vi "Resistance Configuration.vi"(8 "error in (no error)":errorcluster, 10 "Resistance Range":T1, 11 "VISA resource name":refnum<visa-resource-name>) -> (0 "error out":errorcluster, 3 "VISA resource name out":refnum<visa-resource-name>)   [LabVIEW 2015, in "Keysight U1252.lvlib"]
uses:
  <instrlib>/Keysight U1252/Keysight U1252.lvlib
  <instrlib>/Keysight U1252/Controls/Resistance Range.ctl
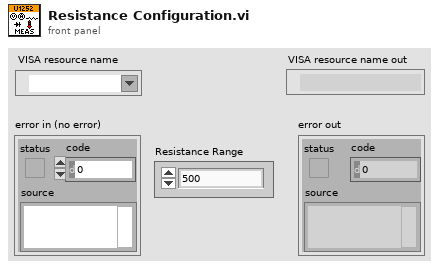
[diagram p1: front panel]
types:
  T1 = typedef "Keysight U1252.lvlib/Resistance Range.ctl" = enum16{"500", "5k", "50k", "500k", "5M", "50M", "500M", "Auto"}
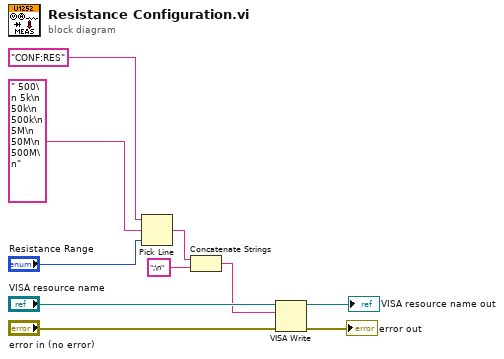
[diagram p0: block diagram]
diagram:
  n1 = Pick Line(string ("")="CONF:RES", multi-line string=" 500\n 5k\n 50k\n 500k\n 5M\n 50M\n 500M\n", line index="Resistance Range") -> (output string=w4:string)
  n2 = Concatenate Strings(w4, ";\n" ("string")) -> (w2:string)
  n3 = VISA Write(VISA resource name="VISA resource name", write buffer=w2, error in (no error)="error in (no error)") -> (VISA resource name out=→"VISA resource name out":refnum<visa-resource-name>, error out=→"error out":errorcluster)  [unwired: 1 out]
